vi "F.vi"(9 "Z":u32 format="%08x", 10 "Y":u32 format="%08x", 11 "X":u32 format="%08x") -> (3 "F":u32 format="%08x")   [LabVIEW 2013, in "MD5.lvlib" / "MD5.lvclass"]
uses:
  MD5.lvclass
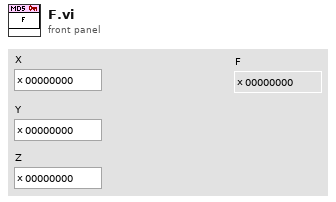
[diagram p1: front panel]
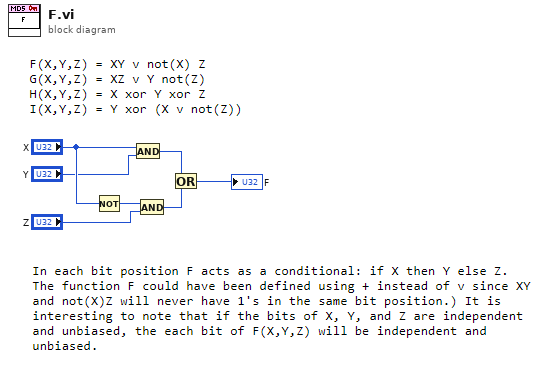
[diagram p0: block diagram]
diagram:
  n1 = Not(x="X") -> (.not. x?=w7:u32)
  n2 = And(x="X", y="Y") -> (x .and. y?=w3:u32)
  n3 = And(x=w7, y="Z") -> (x .and. y?=w2:u32)
  n4 = Or(x=w3, y=w2) -> (x .or. y?=→"F":u32)
